vi "Get Control Information.vi"(8 "error in (no error)":errorcluster, 11 "Cluster in":refnum<class "Cluster.lvclass">) -> (0 "error out":errorcluster, 2 "Control Information":string[][](array[string]), 3 "Cluster out":refnum<class "Cluster.lvclass">)   [LabVIEW 2017, in "Localization.lvlib" / "Cluster.lvclass"]
doc: "VI for override that is supposed to do go throgh the process for each control type and pull out the information that is necessary for each control.\n\nChoose Movement Consulting, LLC"
uses:
  Cluster.lvclass
  C:/Apps/CMC/OpenSource/Localization/Control Info/Control Info.lvclass
  Control Info/Control Info.lvclass
  Localization.lvlib
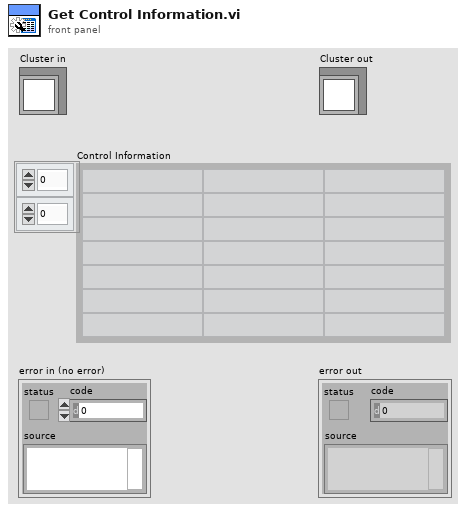
[diagram p1: front panel]
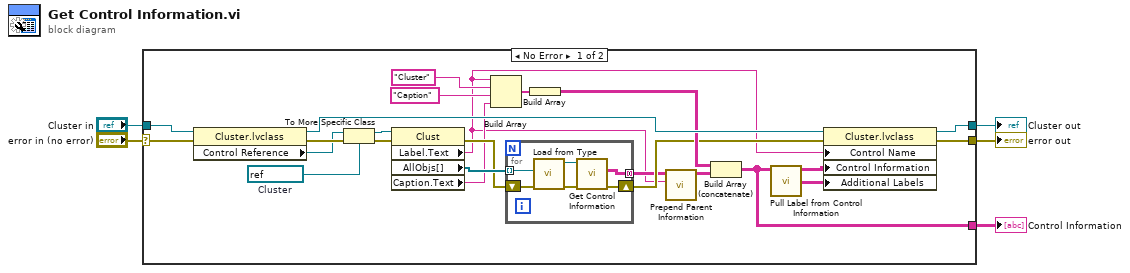
[diagram p0: block diagram]
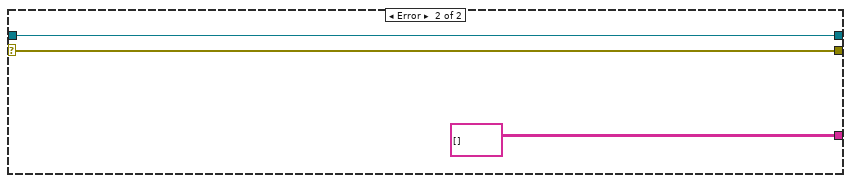
[diagram p2: hidden frame]
diagram:
  n1 = case shown="No Error" "error in (no error)" {
    selector: "error in (no error)" -> [w24 w38]
    tunnel: [w21 w38] -> w2
    tunnel: "Cluster in" -> [w23 w37]
    tunnel: [w8 string[][] []] -> w3
    tunnel: [w19 w37] -> w1
    frame No Error {
      w29 = refnum<vi> refnum  # Cluster
      n2 = property class="Cluster.lvclass"(reference=w23, error in=w24) -> (reference out=w20:refnum<class "Cluster.lvclass">, error out=w25:errorcluster, "Control Reference"=w22:refnum<vi>)
      n3 = To More Specific Class(target class=w29, reference=w22, error in=w25) -> (specific class reference=w28:refnum<vi>, error out=w26:errorcluster)
      n4 = property class="Clust"(reference=w28, error in=w26) -> (error out=w14:errorcluster, "Label.Text"=w9:string, "AllObjs[]"=w16:refnum<vi>[], "Caption.Text"=w10:string)  [unwired: 1 out]
      n5 = Build Array(w9, "Cluster", "Caption", w10) -> (w27:string[])
      n6 = for {
        tunnel: w16 -> [w35] mode=indexing
        shift-right: [w31] -> w13
        shift-left: w14 -> [w34]
        tunnel: [w30] -> w12 mode=concatenating
        n7 = call "Load from Type.vi"("error in (no error)"=w34, "Control Reference"=w35) -> ("error out"=w32:errorcluster, "Control Info out"=w33:refnum<class "Control Info.lvclass">)  [unwired: 8 in]
        n8 = call-dynamic "Get Control Information.vi"("error in (no error)"=w32, "Control Info in"=w33) -> ("error out"=w31:errorcluster, "Control Information"=w30:string[][])  [unwired: 7 in, 1 out]
      }
      n9 = Build Array(w27) -> (w15:string[][])
      n10 = call "Prepend Parent Information.vi"("Prepend String"=w9, "Control Information in"=w12) -> ("Control Information out"=w11:string[][])  [unwired: 9 in]
      n11 = Build Array (concatenate)(w15, w11) -> (w8:string[][])
      n12 = call "Pull Label from Control Information.vi"("Control Caption Table"=w8) -> ("Additional Labels"=w6:string[][], "Control Information"=w7:string[][])  [unwired: 9 in]
      n13 = property class="Cluster.lvclass"(reference=w20, error in=w13, "Control Name"=w9, "Control Information"=w7, "Additional Labels"=w6) -> (reference out=w19:refnum<class "Cluster.lvclass">, error out=w21:errorcluster)
    }
    frame Error {
    }
  }
  "error out" <- w2
  "Cluster out" <- w1
  "Control Information" <- w3
